vi "Initialize HW.vi"(8 "error in (no error)":errorcluster, 11 "DAQmx Switch in":refnum<class "DAQmx Switch.lvclass">) -> (0 "error out":errorcluster, 3 "DAQmx Switch out":refnum<class "DAQmx Switch.lvclass">)   [LabVIEW 2020, in "DAQmx Switch.lvclass"]
uses:
  DAQmx Switch.lvclass
  DAQmx Switch.lvclass/DAQmx Switch.ctl
  <vilib>/DAQmx/create/channels.llb/DAQmx Create Channel (DO-Digital Output).vi
  Switch.lvclass
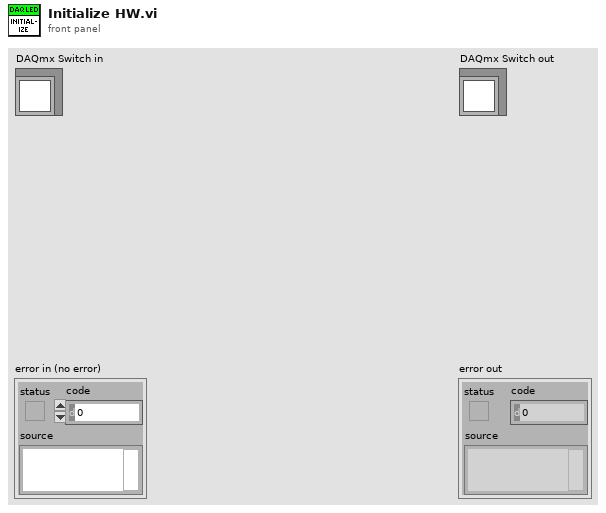
[diagram p1: front panel]
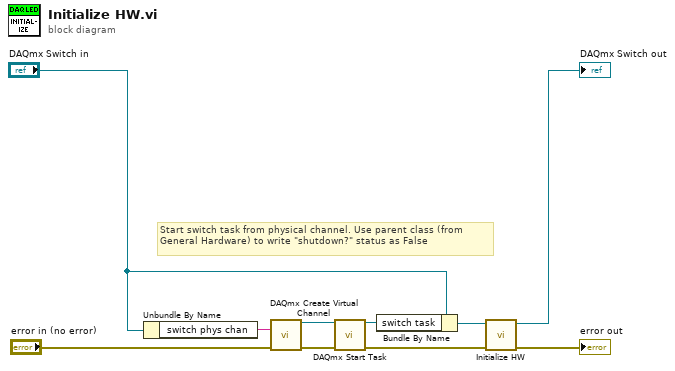
[diagram p0: block diagram]
diagram:
  # "Start switch task from physical channel. Use parent class (from General Hardware) to write \"shutdown?\" status as False"
  n1 = Unbundle By Name("DAQmx Switch in") -> ("switch phys chan"=w9:tag)
  n2 = call-poly <vilib>:"DAQmx Create Virtual Channel.vi"("lines"=w9, "error in"="error in (no error)") -> ("task out"=w5:refnum<k21>, "error out"=w7:errorcluster)  [unwired: 12 in]
  n3 = call <vilib>:"DAQmx Start Task.vi"("task/channels in"=w5, "error in"=w7) -> ("task out"=w3:refnum<k21>, "error out"=w6:errorcluster)  [unwired: 12 in]
  n4 = Bundle By Name(cluster="DAQmx Switch in", "switch task"=w3) -> (w2:refnum<class "DAQmx Switch.lvclass">)
  n5 = call-parent "Initialize HW.vi"("error in (no error)"=w6, "Switch in"=w2) -> ("error out"=→"error out":errorcluster, "Switch out"=→"DAQmx Switch out":refnum<class "DAQmx Switch.lvclass">)  [unwired: 8 in]
